vi "Destroy.vi"(8 "error in":errorcluster, 11 "BigMAQ in":refnum<class "BigMAQ.lvclass">) -> (0 "error out":errorcluster, 3 "BigMAQ out":refnum<class "BigMAQ.lvclass">)   [LabVIEW 2019, in "BigMAQ.lvclass"]
uses:
  BigMAQ.lvclass
  <vilib>/vision/Image Controls.llb/IMAQ Image.ctl
  BigMAQ.lvclass/BigMAQ.ctl
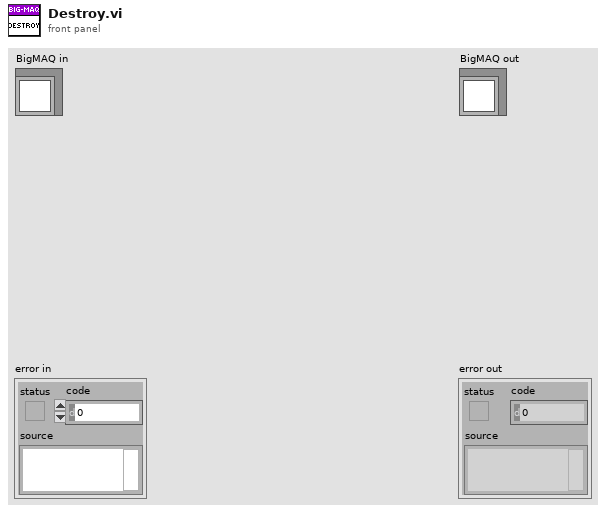
[diagram p1: front panel]
types:
  T1 = typedef "IMAQ Image.ctl" = refnum<image>
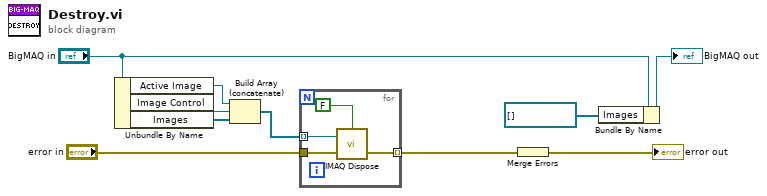
[diagram p0: block diagram]
diagram:
  n1 = Unbundle By Name("BigMAQ in") -> ("Active Image"=w1:T1, "Image Control"=w5:T1, "Images"=w4:T1[])
  n2 = Build Array (concatenate)(w1, w5, w4) -> (w3:T1[])
  n3 = for {
    tunnel: w3 -> [w13] mode=indexing
    tunnel: "error in" -> [w12]
    tunnel: [w11] -> w9 mode=indexing
    n4 = call "IMAQ Dispose"("All Images? (No)"=FALSE, "Image"=w13, "error in (no error)"=w12) -> ("error out"=w11:errorcluster)  [unwired: 3 in]
  }
  n5 = Merge Errors(w9) -> (→"error out":errorcluster)
  n6 = Bundle By Name(cluster="BigMAQ in", "Images"=T1[] []) -> (→"BigMAQ out":refnum<class "BigMAQ.lvclass">)
